vi "pf Get Property Info.vi"(8 "error in (no error)":errorcluster, 10 "iProperty":i32, 11 "iPort":i32) -> (0 "error out":errorcluster, 1 "iPropFlag":i32, 2 "iPropType":i32, 3 "function return":string)   [LabVIEW 2025, in "Photonfocus_Toolkit.lvlib"]
doc: "PFCONFIG_API const char* pfGetPropertyInfo(int iProperty);"
uses:
  Photonfocus_Toolkit.lvlib
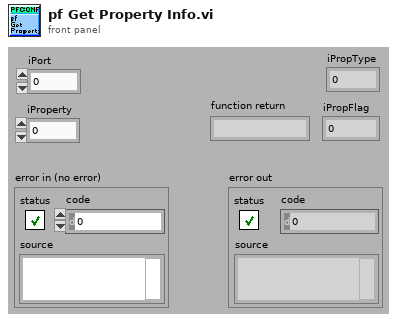
[diagram p1: front panel]
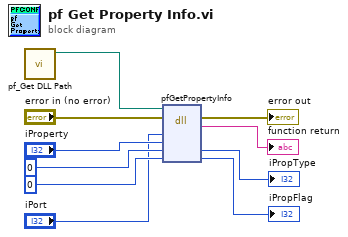
[diagram p0: block diagram]
diagram:
  n1 = call "pf_Get DLL Path.vi"() -> ("DLL path"=w7:path)  [unwired: 1 in, 10 out]
  n2 = dll-call lib="S:/Progetti/Photonfocus/Codice/DEV/PFConfig_lvlib/PFConfig.*" fn="pfGetPropertyInfo"(path in=w7, error in="error in (no error)", "iPort"="iPort", "iProperty"="iProperty", "iPropType"=0, "iPropFlag"=0) -> (error out=→"error out":errorcluster, "return type"=→"function return":string, "iPropType"=→"iPropType":i32, "iPropFlag"=→"iPropFlag":i32)  [unwired: 3 in, 1 out]
